vi "Who is the winner.vi"() -> ()   [LabVIEW 2020]
panel:
  out "stop 2":bool
  in  "Select Season":bool
  in  "Select League":bool
  in  "Select Country":bool
  in  "Contine":bool
  out "String":string
  out "error out":errorcluster
  in  "error in (no error)":errorcluster
  in  "stop":bool
  in  "Season":u16(ring) items=["2020-09-18", "2019-08-16", "2018-08-24", "2017-08-18", "2016-08-26", "2015-08-14", "2014-08-22", "2013-08-09", "2012-08-24", "2011-08-05", "2010-08-20", "2009-08-07", "2008-08-15", "2007-08-10", "2006-08-11", "2005-08-05", "2004-08-06", "2003-08-01", "2002-08-09", "2001-07-28", "2000-08-11", "1999-08-13", "1998-08-14", "1997-08-01", "1996-08-16", "1995-08-09", "1994-08-17", "1993-08-05", "1992-08-12", "1991-07-31", "1990-08-06", "1989-07-26", "1988-07-20", "1987-07-29", "1986-08-06", "1985-08-07", "1984-08-22", "1983-08-10", "1982-08-15", "1981-08-06", "1980-08-13", "1979-08-09", "1978-08-09", "1977-08-04", "1976-08-12", "1975-08-07", "1974-08-22", "1973-07-23", "1972-09-14", "1971-08-12", "1970-08-13", "1969-08-14", "1968-08-15", "1967-08-16", "1966-08-18", "1965-07-23", "1964-08-20", "1963-08-23"]
  in  "League":u16(ring) items=["DFB-Pokal", "Regionalliga", "3. Liga", "2. Bundesliga", "Bundesliga", "Frauen Bundesliga", "DFL Super Cup"]
  out "Numeric":i32
  in  "Country":u16(ring) items=["Africa", "Argentina", "Asia", "Australia", "Austria", "Belgium", "Bolivia", "Bosnia and Herzegovina", "Brazil", "Bulgaria", "Canada", "Chile", "China PR", "Colombia", "Croatia", "Czech Republic", "Denmark", "Ecuador", "England", "Estonia", "Europe", "Finland", "France", "Germany", "Greece", "Hungary", "Iceland", "India", "Israel", "Italy", "Japan", "Latvia", "Lithuania", "Malta", "Mexico", "Netherlands", "Northern Ireland", "Norway", "Oceania", "Panama", "Peru", "Poland", "Portugal", "Republic of Ireland", "Romania", "Russia", "Scotland", "South Africa", "South America", "Spain", "Sweden", "Switzerland", "Turkey", "Ukraine", "United States", "Uruguay", "Venezuela", "Vietnam", "Wales", "World"]
  out "Info":string
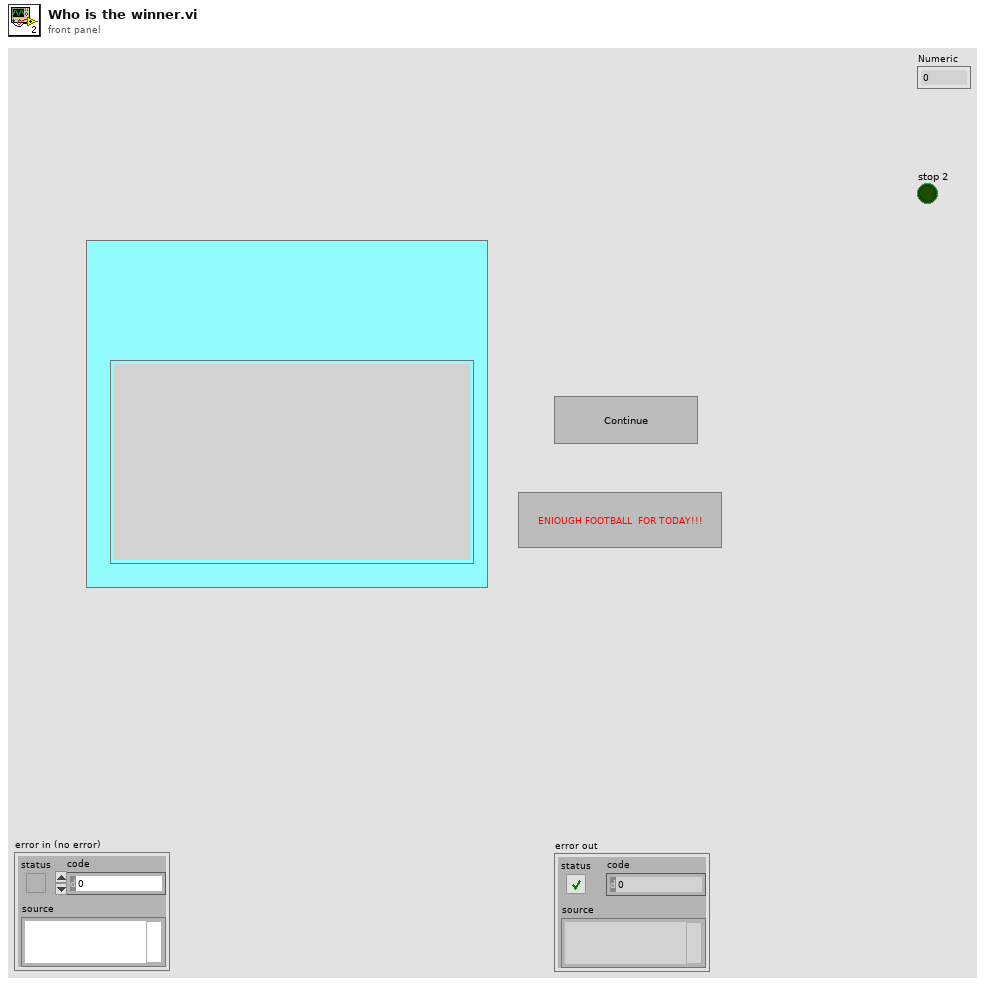
[diagram p1: front panel]
types:
  T1 = cluster{"id":i32, "startDate":string, "endDate":string, "winner":cluster{"name":string, "crestUrl":string, "shortName":string}}[]
  T2 = cluster{"count":i32, "competitions":cluster{"id":i32, "code":string, "name":string, "area":cluster{"name":string, "id":i32, "countryCode":string}, "currentSeason":cluster{"startDate":string, "endDate":string, "currentMatchday":i32}}[]}
  T3 = cluster{"id":i32, "code":string, "name":string, "area":cluster{"name":string, "id":i32, "countryCode":string}, "currentSeason":cluster{"startDate":string, "endDate":string, "currentMatchday":i32}}[]
  T4 = cluster{"id":i32, "area":cluster{"name":string}, "name":string, "code":string, "currentSeason":cluster{"startDate":string, "endDate":string, "currentMatchday":i32, "winner":string}, "seasons":cluster{"id":i32, "startDate":string, "endDate":string, "winner":cluster{"name":string, "crestUrl":string, "shortName":string}}[]}
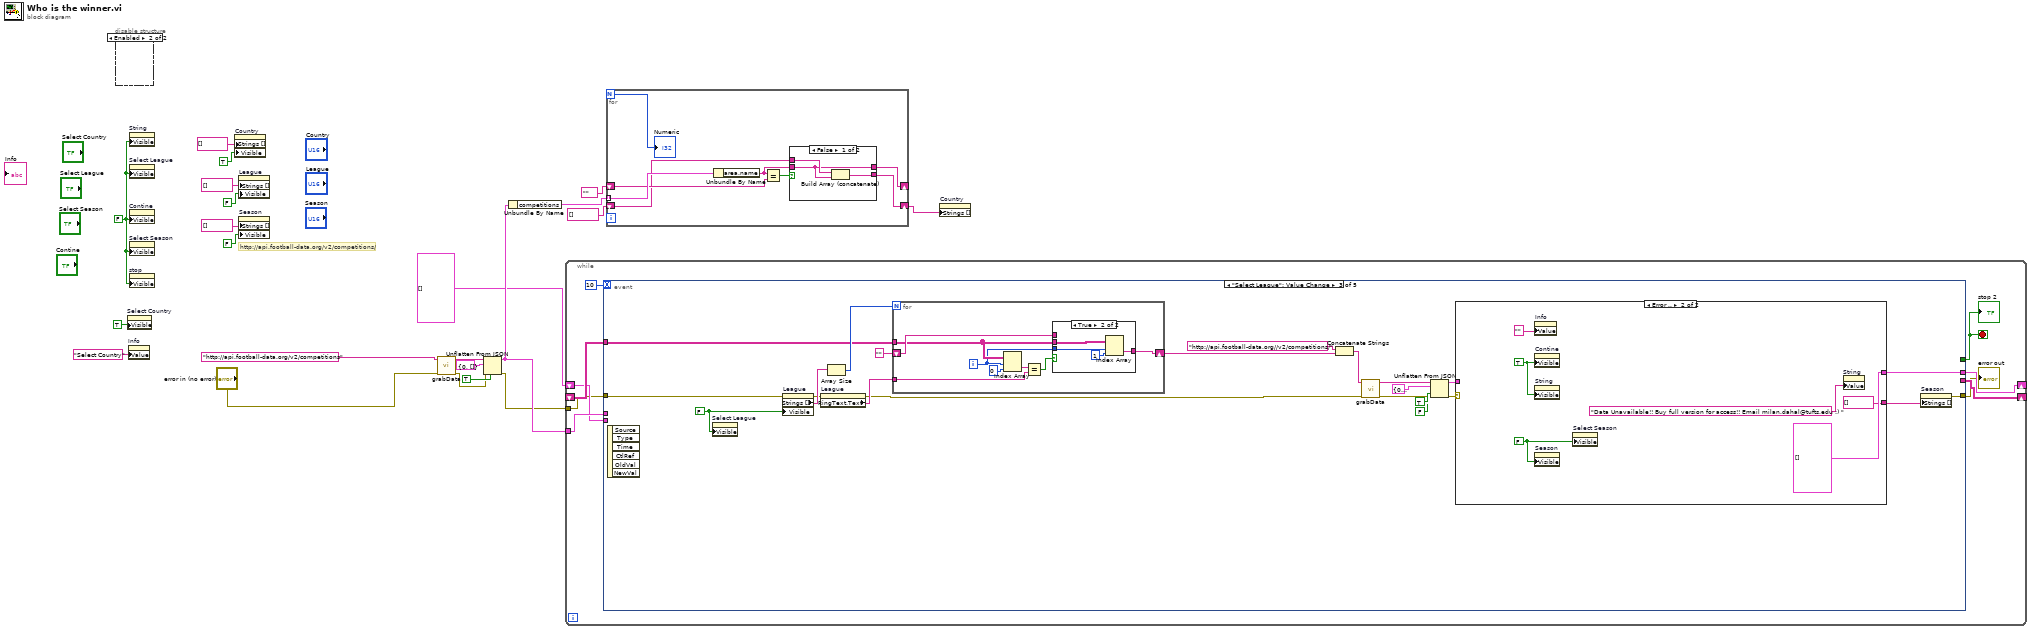
[diagram p0: block diagram]
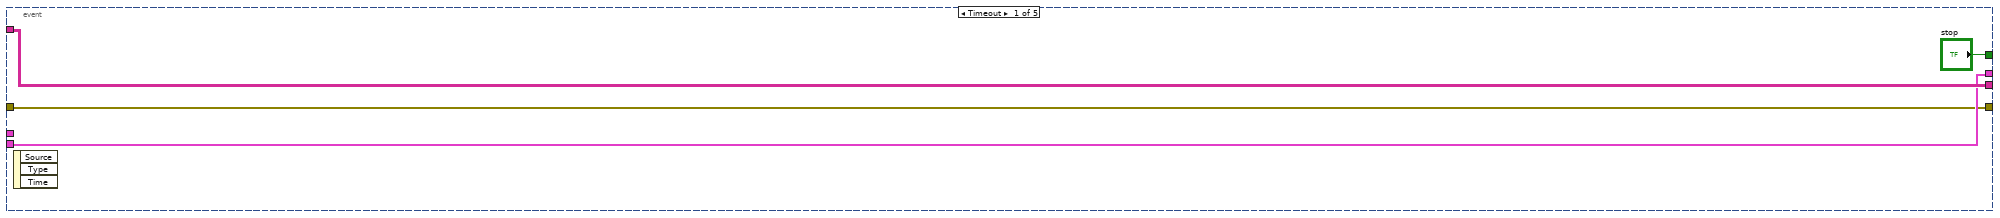
[diagram p2: hidden frame]
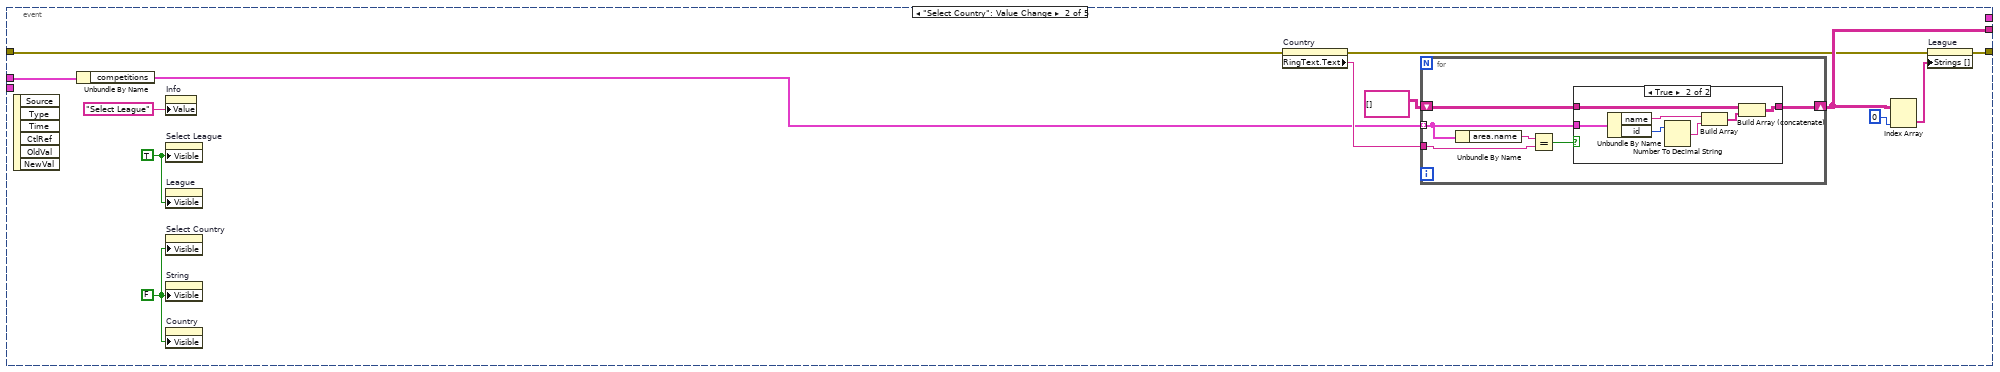
[diagram p3: hidden frame]
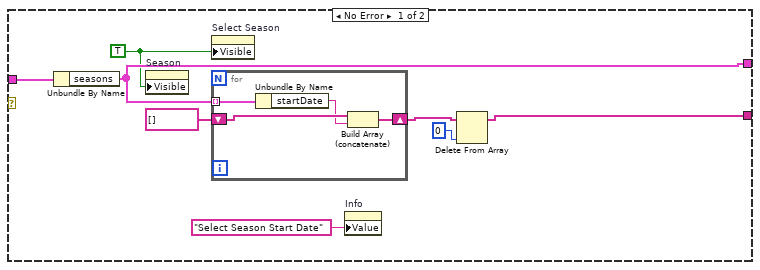
[diagram p5: hidden frame]
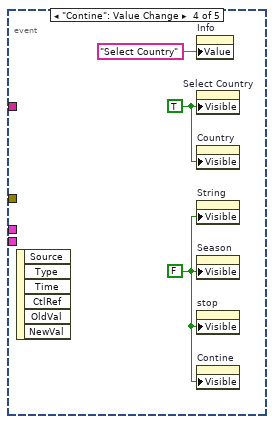
[diagram p7: hidden frame]
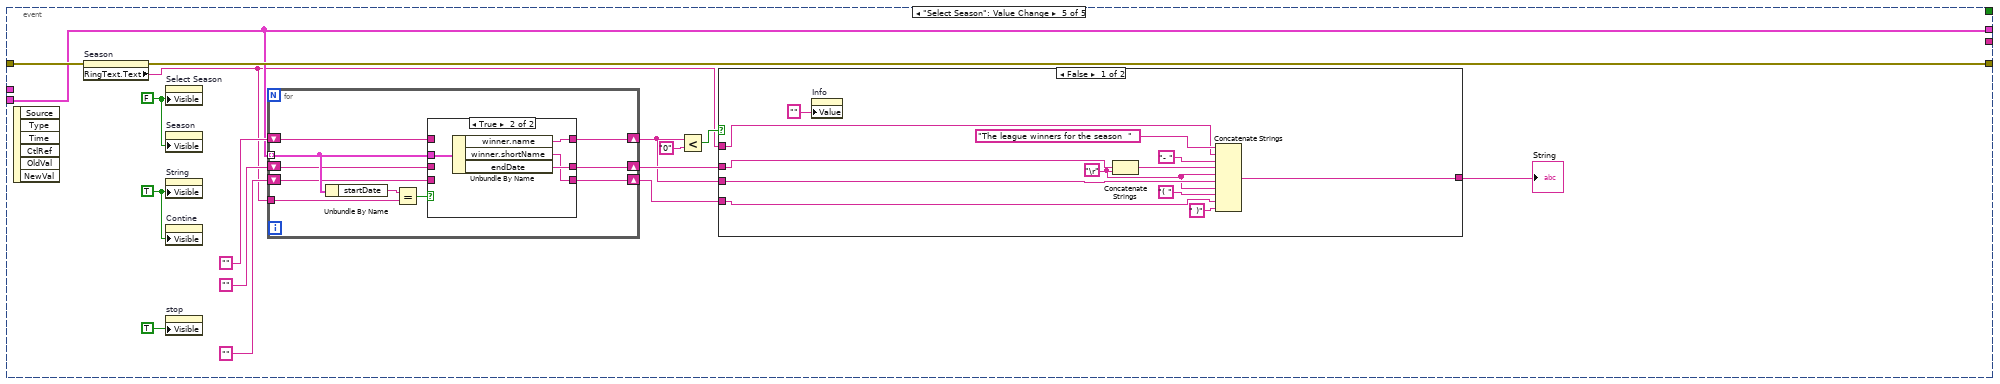
[diagram p8: hidden frame]
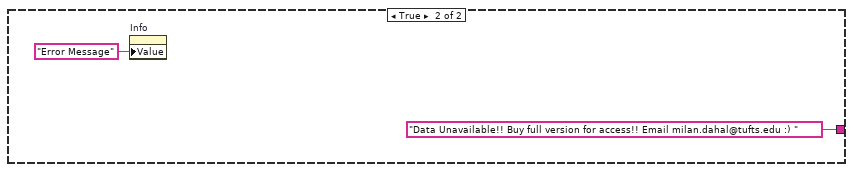
[diagram p9: hidden frame]
diagram:
  w2 = FALSE ("Visible")
  # "http://api.football-data.org/v2/competitions/"
  n1 = disable-structure shown="Enabled" {
    frame Disabled {
    }
    frame Enabled {
    }
  }
  n2 = property on="Select Country" class="Bool"("Visible"=TRUE) -> ()  [unwired: 2 in, 2 out]
  n3 = property on="Info" class="Str"("Value"="Select Country" ("Info")) -> ()  [unwired: 2 in, 2 out]
  n4 = property on="String" class="Str"("Visible"=w2) -> ()  [unwired: 2 in, 2 out]
  n5 = property on="Select League" class="Bool"("Visible"=w2) -> ()  [unwired: 2 in, 2 out]
  n6 = property on="Contine" class="Bool"("Visible"=w2) -> ()  [unwired: 2 in, 2 out]
  n7 = property on="Select Season" class="Bool"("Visible"=w2) -> ()  [unwired: 2 in, 2 out]
  n8 = property on="stop" class="Bool"("Visible"=w2) -> ()  [unwired: 2 in, 2 out]
  n9 = property on="Country" class="Ring (strict)"("Strings []"=string[] [], "Visible"=TRUE) -> ()  [unwired: 2 in, 2 out]
  n10 = property on="League" class="Ring (strict)"("Strings []"=string[] [], "Visible"=FALSE) -> ()  [unwired: 2 in, 2 out]
  n11 = property on="Season" class="Ring (strict)"("Strings []"=string[] [], "Visible"=FALSE) -> ()  [unwired: 2 in, 2 out]
  n12 = call "grabData.vi"("error in (no error)"="error in (no error)", "URL"="http://api.football-data.org/v2/competitions" ("url")) -> ("error out"=w11:errorcluster, "body"=w22:string)  [unwired: 8 in]
  n13 = Unflatten From JSON(JSON string=w22, type and defaults=T2 {"count"=0, "competitions"=[]}, default null elements? (F)=TRUE, error in (no error)=w11) -> (value=w15:T2, error out=w10:errorcluster)  [unwired: 3 in]
  n14 = Unbundle By Name(w15) -> ("competitions"=w19:T3)
  n15 = while {
    shift-right: [w29] -> _
    shift-left: _ -> [w31]
    tunnel: w15 -> [w30]
    shift-right: [w28] -> _
    shift-left: T1 [] ("seasons") -> [w27]
    tunnel: w10 -> [w26]
    stop <- w24 stop-if-true
    n16 = event shown="[2] \"Select League\": Value Change" {
      selector: _ -> [_ _ _ _ _]
      dyn-events: _ -> [_ _ _ _ _]
      timeout: 10 -> [_ _ _ _ _]
      tunnel: w31 -> [w35 _ w76 _ _]
      tunnel: [w35 w43 _ _ _] -> w29
      tunnel: w30 -> [_ w44 _ _ _]
      tunnel: [w34 _ w63 _ w130] -> w28
      tunnel: w27 -> [w34 _ _ _ w130]
      tunnel: w26 -> [w33 w41 w73 _ w132]
      tunnel: [w33 w39 w69 _ w131] -> w25
      tunnel: ["stop" _ _ _ _] -> w24
      event Timeout {
        n17 = event-data() -> ()  [unwired: 1 in, 3 out]
      }
      event "Select Country": Value Change {
        w37 = FALSE ("Visible")
        w38 = TRUE ("Visible")
        n18 = event-data() -> ()  [unwired: 1 in, 6 out]
        n19 = Unbundle By Name(w44) -> ("competitions"=w46:T3)
        n20 = property on="Info" class="Str"("Value"="Select League" ("Info")) -> ()  [unwired: 2 in, 2 out]
        n21 = property on="Select League" class="Bool"("Visible"=w38) -> ()  [unwired: 2 in, 2 out]
        n22 = property on="League" class="Ring (strict)"("Visible"=w38) -> ()  [unwired: 2 in, 2 out]
        n23 = property on="Select Country" class="Bool"("Visible"=w37) -> ()  [unwired: 2 in, 2 out]
        n24 = property on="String" class="Str"("Visible"=w37) -> ()  [unwired: 2 in, 2 out]
        n25 = property on="Country" class="Ring (strict)"("Visible"=w37) -> ()  [unwired: 2 in, 2 out]
        n26 = property on="Country" class="Ring (strict)"(error in=w41) -> (error out=w40:errorcluster, "RingText.Text"=w47:string)  [unwired: 1 in, 1 out]
        n27 = for {
          tunnel: w46 -> [w50] mode=indexing
          shift-right: [w49] -> w43
          shift-left: string[][] [] -> [w52]
          tunnel: w47 -> [w51]
          n28 = Unbundle By Name(w50) -> ("area.name"=w53:string)
          n29 = Equal?(x=w53, y=w51) -> (x = y?=w54:bool)
          n30 = case shown="True" w54 {
            tunnel: w52 -> [w55 w61]
            tunnel: [w55 w60] -> w49
            tunnel: w50 -> [_ w62]
            frame False {
            }
            frame True {
              n31 = Unbundle By Name(w62) -> ("name"=w58:string, "id"=w59:i32)
              n32 = Number To Decimal String(number=w59) -> (decimal integer string=w57:string)  [unwired: 1 in]
              n33 = Build Array(w58, w57) -> (w56:string[])
              n34 = Build Array (concatenate)(w61, w56) -> (w60:string[][])
            }
          }
        }
        n35 = Index Array(array=w43, index (col)=0 ("disabled index (col)")) -> (element=w48:string[])  [unwired: 1 in]
        n36 = property on="League" class="Ring (strict)"(error in=w40, "Strings []"=w48) -> (error out=w39:errorcluster)  [unwired: 1 in, 1 out]
      }
      event "Select League": Value Change {
        w68 = FALSE ("Visible")
        n37 = event-data() -> ()  [unwired: 1 in, 6 out]
        n38 = property on="Select League" class="Bool"("Visible"=w68) -> ()  [unwired: 2 in, 2 out]
        n39 = property on="League" class="Ring (strict)"(error in=w73, "Visible"=w68) -> (error out=w72:errorcluster, "Strings []"=w84:string[])  [unwired: 1 in, 1 out]
        n40 = property on="League" class="Ring (strict)"(error in=w72) -> (error out=w71:errorcluster, "RingText.Text"=w81:string)  [unwired: 1 in, 1 out]
        n41 = Array Size(array=w84) -> (size(s)=w83:i32)
        n42 = for {
          N: w83 -> [_]
          tunnel: w76 -> [w107]
          shift-right: [w108] -> w82
          shift-left: "" -> [w110]
          tunnel: w81 -> [w109]
          i -> [w103]
          n43 = Index Array(array=w107, index (row)=w103, index (col)=0 ("disabled index (col)")) -> (element=w106:string)
          n44 = Equal?(x=w106, y=w109) -> (x = y?=w104:bool)
          n45 = case shown="True" w104 {
            tunnel: w110 -> [w111 _]
            tunnel: [w111 w114] -> w108
            tunnel: w107 -> [_ w115]
            tunnel: w103 -> [_ w112]
            frame False {
            }
            frame True {
              n46 = Index Array(array=w115, index (row)=w112, index (col)=1 ("disabled index (col)")) -> (element=w114:string)
            }
          }
        }
        n47 = Concatenate Strings("http://api.football-data.org//v2/competitions/" ("url"), w82) -> (w75:string)
        n48 = call "grabData.vi"("error in (no error)"=w71, "URL"=w75) -> ("error out"=w70:errorcluster, "body"=w74:string)  [unwired: 8 in]
        n49 = Unflatten From JSON(JSON string=w74, type and defaults=T4 {"id"=0, "area"={"name"=""}, "name"="", "code"="", "currentSeason"={"startDate"="", "endDate"="", "currentMatchday"=0, "winner"=""}, "seasons"=[]}, default null elements? (F)=TRUE, strict validation? (F)=FALSE, error in (no error)=w70) -> (value=w65:T4, error out=w66:errorcluster)  [unwired: 2 in]
        n50 = case shown="Error .." w66 {
          tunnel: w65 -> [w91 _]
          tunnel: [w87 string[] []] -> w64
          tunnel: [w90 T1 [] ("seasons")] -> w63
          frame No Error {
            w89 = TRUE ("Visible")
            n51 = Unbundle By Name(w91) -> ("seasons"=w90:T1)
            n52 = property on="Season" class="Ring (strict)"("Visible"=w89) -> ()  [unwired: 2 in, 2 out]
            n53 = property on="Select Season" class="Bool"("Visible"=w89) -> ()  [unwired: 2 in, 2 out]
            n54 = for {
              tunnel: w90 -> [w96] mode=indexing
              shift-right: [w93] -> w88
              shift-left: string[] [] -> [w95]
              n55 = Unbundle By Name(w96) -> ("startDate"=w94:string)
              n56 = Build Array (concatenate)(w95, w94) -> (w93:string[])
            }
            n57 = property on="Info" class="Str"("Value"="Select Season Start Date" ("Info")) -> ()  [unwired: 2 in, 2 out]
            n58 = Delete From Array(array=w88, index=0) -> (array with subset deleted=w87:string[])  [unwired: 1 in, 1 out]
          }
          frame Error {
            w100 = FALSE ("Visible")
            w98 = TRUE ("Visible")
            n59 = property on="Info" class="Str"("Value"="" ("Info")) -> ()  [unwired: 2 in, 2 out]
            n60 = property on="Contine" class="Bool"("Visible"=w98) -> ()  [unwired: 2 in, 2 out]
            n61 = property on="String" class="Str"("Visible"=w98) -> ()  [unwired: 2 in, 2 out]
            n62 = property on="Season" class="Ring (strict)"("Visible"=w100) -> ()  [unwired: 2 in, 2 out]
            n63 = property on="Select Season" class="Bool"("Visible"=w100) -> ()  [unwired: 2 in, 2 out]
            n64 = property on="String" class="Str"("Value"="Data Unavailable!! Buy full version for access!! Email milan.dahal@tufts.edu :) ") -> ()  [unwired: 2 in, 2 out]
          }
        }
        n65 = property on="Season" class="Ring (strict)"("Strings []"=w64) -> (error out=w69:errorcluster)  [unwired: 2 in, 1 out]
      }
      event "Contine": Value Change {
        w117 = FALSE ("Visible")
        w118 = TRUE ("Visible")
        n66 = event-data() -> ()  [unwired: 1 in, 6 out]
        n67 = property on="Info" class="Str"("Value"="Select Country" ("Info")) -> ()  [unwired: 2 in, 2 out]
        n68 = property on="Select Country" class="Bool"("Visible"=w118) -> ()  [unwired: 2 in, 2 out]
        n69 = property on="Country" class="Ring (strict)"("Visible"=w118) -> ()  [unwired: 2 in, 2 out]
        n70 = property on="String" class="Str"("Visible"=w117) -> ()  [unwired: 2 in, 2 out]
        n71 = property on="Season" class="Ring (strict)"("Visible"=w117) -> ()  [unwired: 2 in, 2 out]
        n72 = property on="stop" class="Bool"("Visible"=w117) -> ()  [unwired: 2 in, 2 out]
        n73 = property on="Contine" class="Bool"("Visible"=w117) -> ()  [unwired: 2 in, 2 out]
      }
      event "Select Season": Value Change {
        w120 = FALSE ("Visible")
        w121 = TRUE ("Visible")
        n74 = event-data() -> ()  [unwired: 1 in, 6 out]
        n75 = property on="Season" class="Ring (strict)"(error in=w132) -> (error out=w131:errorcluster, "RingText.Text"=w125:string)  [unwired: 1 in, 1 out]
        n76 = property on="Select Season" class="Bool"("Visible"=w120) -> ()  [unwired: 2 in, 2 out]
        n77 = property on="Season" class="Ring (strict)"("Visible"=w120) -> ()  [unwired: 2 in, 2 out]
        n78 = property on="String" class="Str"("Visible"=w121) -> ()  [unwired: 2 in, 2 out]
        n79 = property on="Contine" class="Bool"("Visible"=w121) -> ()  [unwired: 2 in, 2 out]
        n80 = property on="stop" class="Bool"("Visible"=TRUE) -> ()  [unwired: 2 in, 2 out]
        n81 = for {
          tunnel: w130 -> [w156] mode=indexing
          shift-right: [w155] -> w123
          shift-left: "" ("crestUrl") -> [w157]
          tunnel: w125 -> [w149]
          shift-right: [w154] -> w124
          shift-left: "" ("endDate") -> [w153]
          shift-right: [w151] -> w122
          shift-left: "" ("shortName") -> [w150]
          n82 = Unbundle By Name(w156) -> ("startDate"=w152:string)
          n83 = Equal?(x=w152, y=w149) -> (x = y?=w158:bool)
          n84 = case shown="True" w158 {
            tunnel: w157 -> [w161 _]
            tunnel: [w161 w164] -> w155
            tunnel: w156 -> [_ w165]
            tunnel: [w160 w163] -> w154
            tunnel: w153 -> [w160 _]
            tunnel: [w159 w162] -> w151
            tunnel: w150 -> [w159 _]
            frame False {
            }
            frame True {
              n85 = Unbundle By Name(w165) -> ("winner.name"=w164:string, "winner.shortName"=w162:string, "endDate"=w163:string)
            }
          }
        }
        n86 = Less?(x=w123, y="0") -> (x < y?=w127:bool)
        n87 = case shown="False" w127 {
          tunnel: [w142 "Data Unavailable!! Buy full version for access!! Email milan.dahal@tufts.edu :) "] -> w126
          tunnel: w125 -> [w145 _]
          tunnel: w124 -> [w138 _]
          tunnel: w123 -> [w143 _]
          tunnel: w122 -> [w140 _]
          frame False {
            w137 = "\r"
            n88 = property on="Info" class="Str"("Value"="" ("Info")) -> ()  [unwired: 2 in, 2 out]
            n89 = Concatenate Strings(w138, w137) -> (w136:string)
            n90 = Concatenate Strings("The league winners for the season  " ("string"), w145, "- " ("string"), w136, w137, w143, w137, "( " ("string"), w140, " )" ("string")) -> (w142:string)
          }
          frame True {
            n91 = property on="Info" class="Str"("Value"="Error Message" ("Info")) -> ()  [unwired: 2 in, 2 out]
          }
        }
        "String" <- w126
      }
    }
    "error out" <- w25
    "stop 2" <- w24
  }
  n92 = for {
    N -> [w166]
    tunnel: w19 -> [w173] mode=indexing
    shift-right: [w169] -> _
    shift-left: "" ("name") -> [w170]
    shift-right: [w167] -> w17
    shift-left: string[] [] -> [w168]
    n93 = Unbundle By Name(w173) -> ("area.name"=w171:string)
    n94 = Equal?(x=w171, y=w170) -> (x = y?=w172:bool)
    n95 = case shown="False" w172 {
      tunnel: w171 -> [w174 w178]
      tunnel: [w174 w178] -> w169
      tunnel: w168 -> [w175 w177]
      tunnel: [w176 w177] -> w167
      frame False {
        n96 = Build Array (concatenate)(w175, w174) -> (w176:string[])
      }
      frame True {
      }
    }
    "Numeric" <- w166
  }
  n97 = property on="Country" class="Ring (strict)"("Strings []"=w17) -> ()  [unwired: 2 in, 2 out]
